vi "mean_baseline.vi"(10 "Mean":dbl, 11 "Ideal Mean":dbl=1600.0) -> (2 "Mean is capacitive":bool, 3 "Mean is conductive":bool)   [LabVIEW 2012]
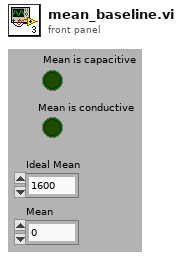
[diagram p1: front panel]
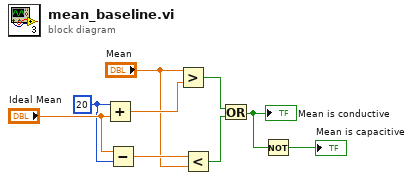
[diagram p0: block diagram]
diagram:
  w7 = 20
  n1 = Add(x=w7, y="Ideal Mean") -> (x+y=w9:dbl)
  n2 = Subtract(x="Ideal Mean", y=w7) -> (x-y=w6:dbl)
  n3 = Greater?(x="Mean", y=w9) -> (0:w4:bool)
  n4 = Less?(x=w6, y="Mean") -> (x < y?=w3:bool)
  n5 = Or(x=w4, y=w3) -> (x .or. y?=w2:bool)
  "Mean is conductive" <- w2
  n6 = Not(x=w2) -> (.not. x?=→"Mean is capacitive":bool)
